vi "AUTON_Choose_File.vi"(10 "Joystick 2 Refnum":string, 11 "Joystick 1 Refnum":string) -> (1 "Auton File":dbl, 2 "Refresh":bool, 3 "Allow Change":bool)   [LabVIEW 2011]
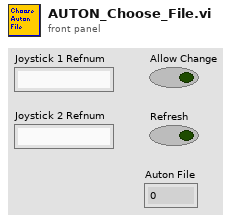
[diagram p1: front panel]
types:
  T1 = typedef "WPI_JoystickDevRef.ctl" = cluster{"Device":T2}
  T2 = typedef "WPI_JoystickDeviceEnum.ctl" = enum16{"USB 1", "USB 2", "USB 3", "USB 4", "Kinect 1", "Kinect 2"}
  T3 = typedef "WPI_JoystickButtonState.ctl" = cluster{"Button 1":bool, "Button 2":bool, "Button 3":bool, "Button 4":bool, "Button 5":bool, "Button 6":bool, "Button 7":bool, "Button 8":bool, "Button 9":bool, "Button 10":bool, "Button 11":bool, "Button 12":bool}
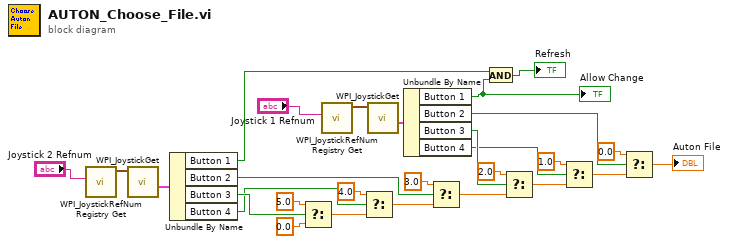
[diagram p0: block diagram]
diagram:
  n1 = call <vilib>:"WPI_JoystickRefNum Registry Get.vi"("refnum name"="Joystick 2 Refnum") -> ("JoystickDevRef"=w6:T1)  [unwired: 9 in, 1 out]
  n2 = call <vilib>:"WPI_JoystickGet.vi"("JoystickDevRef"=w6) -> ("Buttons"=w8:T3)  [unwired: 4 in, 2 out]
  n3 = Unbundle By Name(w8) -> ("Button 1"=w1:bool, "Button 2"=w20:bool, "Button 3"=w26:bool, "Button 4"=w24:bool)
  n4 = Select(t=5.0, s=w26, f=0.0) -> (s? t:f=w25:dbl)
  n5 = call <vilib>:"WPI_JoystickRefNum Registry Get.vi"("refnum name"="Joystick 1 Refnum") -> ("JoystickDevRef"=w3:T1)  [unwired: 9 in, 1 out]
  n6 = Select(t=4.0, s=w24, f=w25) -> (s? t:f=w22:dbl)
  n7 = call <vilib>:"WPI_JoystickGet.vi"("JoystickDevRef"=w3) -> ("Buttons"=w7:T3)  [unwired: 4 in, 2 out]
  n8 = Unbundle By Name(w7) -> ("Button 1"=w2:bool, "Button 2"=w13:bool, "Button 3"=w19:bool, "Button 4"=w18:bool)
  "Allow Change" <- w2
  n9 = Select(t=3.0, s=w20, f=w22) -> (s? t:f=w17:dbl)
  n10 = And(x=w1, y=w2) -> (x .and. y?=→"Refresh":bool)
  n11 = Select(t=2.0, s=w19, f=w17) -> (s? t:f=w11:dbl)
  n12 = Select(t=1.0, s=w18, f=w11) -> (s? t:f=w10:dbl)
  n13 = Select(t=0.0, s=w13, f=w10) -> (s? t:f=→"Auton File":dbl)
